vi "subEventCpp.vi"(8 "error in (no error)":errorcluster, 9 "pathOfOutput":path, 10 "pathOfSubEvent":path, 11 "SalProcess in":refnum<class "SalProcess.lvclass">) -> (0 "error out":errorcluster, 2 "cmd":string, 3 "SalProcess out":refnum<class "SalProcess.lvclass">)   [LabVIEW 2018, in "SalProcess.lvclass"]
doc: "Subscribe the event by CPP."
uses:
  SalProcess.lvclass
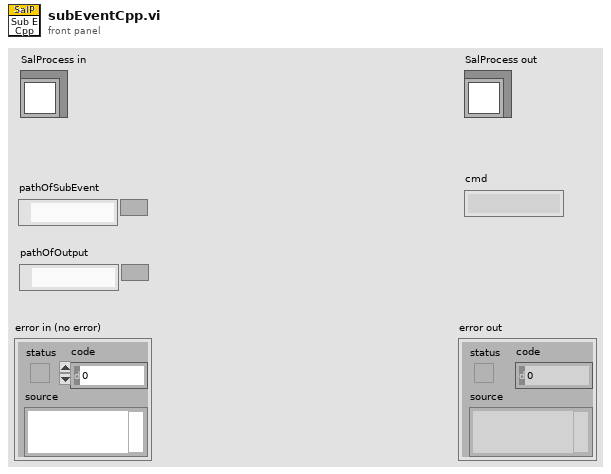
[diagram p1: front panel]
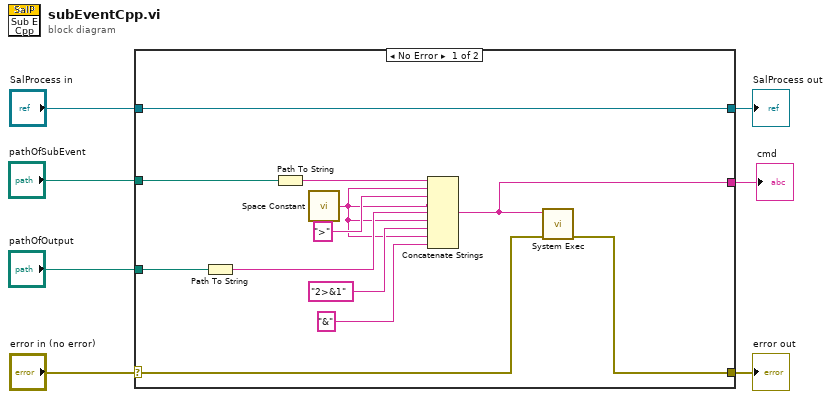
[diagram p0: block diagram]
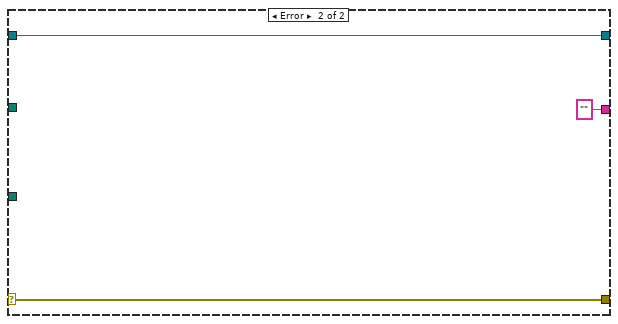
[diagram p2: hidden frame]
diagram:
  n1 = case shown="No Error" "error in (no error)" {
    selector: "error in (no error)" -> [w10 w22]
    tunnel: [w9 w22] -> w6
    tunnel: [w19 w21] -> w4
    tunnel: "SalProcess in" -> [w19 w21]
    tunnel: "pathOfSubEvent" -> [w13 _]
    tunnel: "pathOfOutput" -> [w11 _]
    tunnel: [w8 ""] -> w1
    frame No Error {
      n2 = Path To String(path=w11) -> (string=w17:string)
      n3 = Path To String(path=w13) -> (string=w12:string)
      n4 = call <vilib>:"Space Constant.vi"() -> ("String"=w14:string)
      n5 = Concatenate Strings(w12, w14, ">", w14, w17, w14, "2>&1", w14, "&") -> (w8:string)
      n6 = call <vilib>:"System Exec.vi"("error in (no error)"=w10, "command line"=w8) -> ("error out"=w9:errorcluster)  [unwired: 6 in, 3 out]
    }
    frame Error {
    }
  }
  "error out" <- w6
  "SalProcess out" <- w4
  "cmd" <- w1
